vi "Array of I8_ASCII String To Data.vi"(8 "error in (no error)":errorcluster, 9 "Default":cluster{"I8 Array":i8[]}, 11 "Value":string) -> (0 "error out":errorcluster, 3 "Data":cluster{"I8 Array":i8[]})   [LabVIEW 2010, in "Current Value Table.lvlib"]
doc: "This VI converts data stored on disk as an ascii string into the correct data type. This VI must perform the opposite operation to the DataToASCIIString function."
uses:
  Current Value Table.lvlib
  Errors/Generate Error.vi
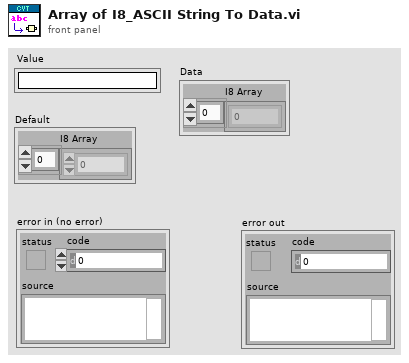
[diagram p1: front panel]
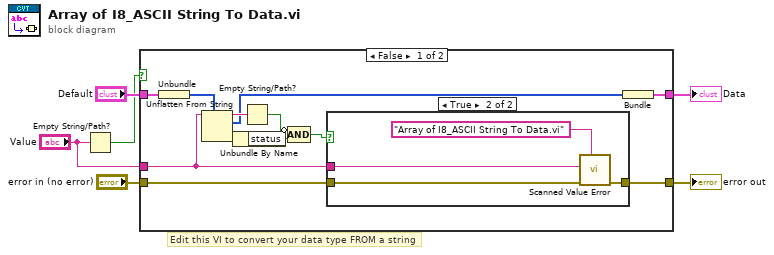
[diagram p0: block diagram]
diagram:
  # "Edit this VI to convert your data type FROM a string"
  n1 = Empty String/Path?(string/path="Value") -> (empty?=w3:bool)
  n2 = case shown="False" w3 {
    tunnel: "Default" -> [w16 w25]
    tunnel: "Value" -> [w12 _]
    tunnel: [w14 w25] -> w1
    tunnel: "error in (no error)" -> [w17 w24]
    tunnel: [w18 w24] -> w5
    frame False {
      n3 = Unbundle(w16) -> ("I8 Array"=w11:i8[])
      n4 = Unflatten From String(type=w11, binary string=w12) -> (rest of the binary string=w9:string, value=w8:i8[], error out=w10:errorcluster)  [unwired: 3 in]
      n5 = Unbundle By Name(w10) -> ("status"=w7:bool)
      n6 = Empty String/Path?(string/path=w9) -> (empty?=w15:bool)
      n7 = Compound Arithmetic op=AND(invert w15, w7) -> (w13:bool)
      n8 = case shown="True" w13 {
        tunnel: [w19 w23] -> w18
        tunnel: w17 -> [w19 w22]
        tunnel: w12 -> [_ w21]
        frame False {
        }
        frame True {
          n9 = call "Scanned Value Error.vi"("caller name"="Array of I8_ASCII String To Data.vi", "error in (no error)"=w22, "Value"=w21) -> ("error out"=w23:errorcluster)  [unwired: 8 in]
        }
      }
      n10 = Bundle("I8 Array"=w8) -> (w14:cluster{"I8 Array":i8[]})  [unwired: 1 in]
    }
    frame True {
    }
  }
  "error out" <- w5
  "Data" <- w1
